vi "sub_vi_arduino_communication.vi"(5 "Cycles":i32, 6 "error in (no error)":errorcluster, 7 "write buffer":string, 9 "VISA resource name in":refnum<visa-resource-name>) -> (0 "error out":errorcluster, 1 "Reads array":dbl[](array[numeric]), 3 "VISA resource name out":refnum<visa-resource-name>, 4 "Received data":string[](array[string]))   [LabVIEW 2016]
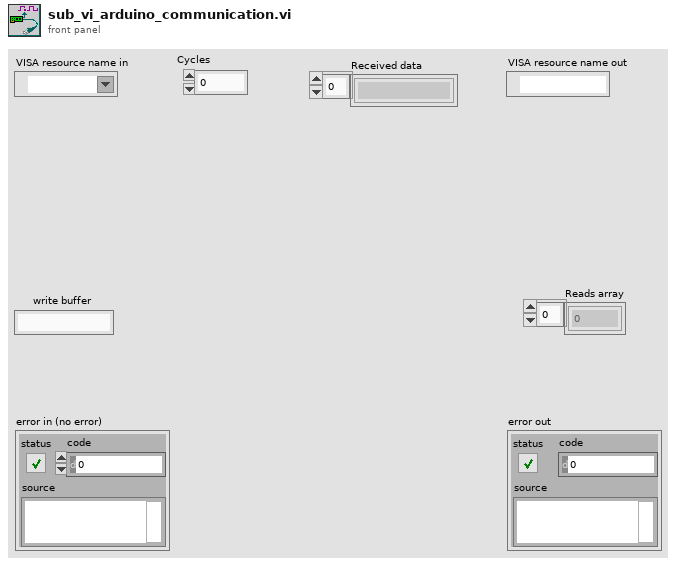
[diagram p1: front panel]
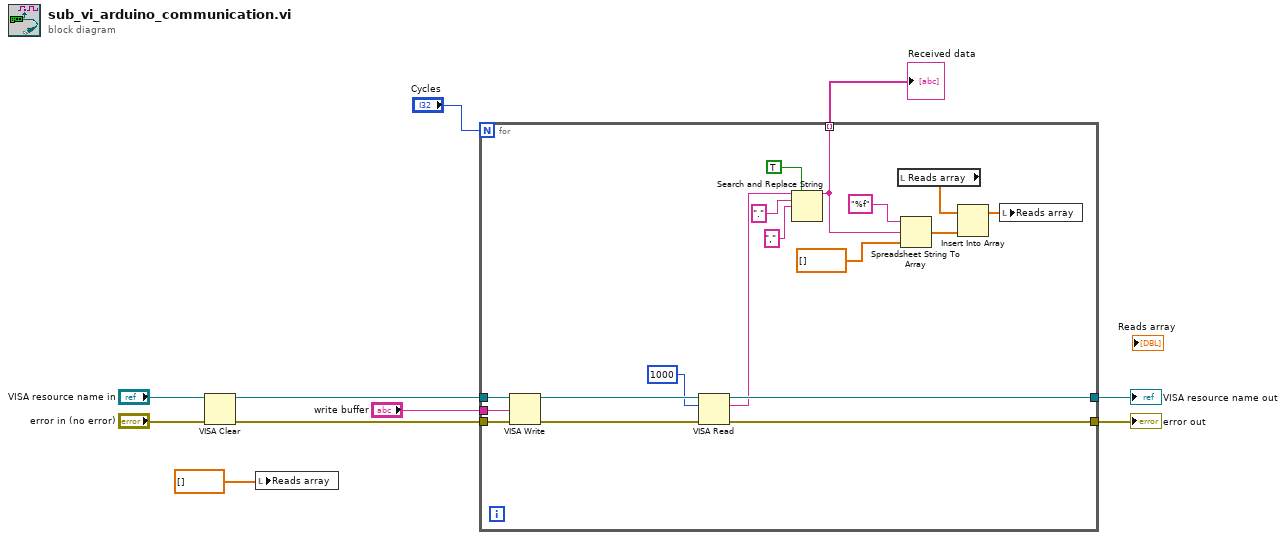
[diagram p0: block diagram]
diagram:
  n1 = VISA Clear(VISA resource name="VISA resource name in", error in (no error)="error in (no error)") -> (VISA resource name out=w6:refnum<visa-resource-name>, error out=w4:errorcluster)
  n2 = local write "Reads array"(dbl[] []) -> ()
  n3 = for {
    N: "Cycles" -> [_]
    tunnel: "write buffer" -> [w26]
    tunnel: w4 -> [w24]
    tunnel: [w28] -> w10
    tunnel: w6 -> [w25]
    tunnel: [w27] -> w9
    tunnel: [w16] -> w2 mode=indexing
    n4 = VISA Write(VISA resource name=w25, write buffer=w26, error in (no error)=w24) -> (VISA resource name out=w22:refnum<visa-resource-name>, error out=w23:errorcluster)  [unwired: 1 out]
    n5 = VISA Read(VISA resource name=w22, byte count=u32 1000, error in (no error)=w23) -> (VISA resource name out=w27:refnum<visa-resource-name>, read buffer=w17:string, error out=w28:errorcluster)  [unwired: 1 out]
    n6 = Search and Replace String(replace all?=TRUE ("replace all? (F)"), input string=w17, search string=".", replace string="," ("replace string (\"\")")) -> (result string=w16:string)  [unwired: 4 in, 3 out]
    n7 = local read "Reads array"() -> (w13:dbl[])
    n8 = Spreadsheet String To Array(format string="%f", spreadsheet string=w16, array type (2D Dbl)=dbl[] []) -> (array=w12:dbl[])  [unwired: 1 in]
    n9 = Insert Into Array(array=w13, new element=w12) -> (w11:dbl[])  [unwired: 1 in]
    n10 = local write "Reads array"(w11) -> ()
  }
  "error out" <- w10
  "VISA resource name out" <- w9
  "Received data" <- w2
